vi "Write Pulse Recorder Configuration.vi"(8 "error in (no error)":errorcluster, 10 "Configuration":T1={"Post-trigger delay"=0.01, "Post-trigger duration"=0.1, "Rate"=1000000.0, "Ranges"=[10.0], "Re-name channels"=[], "Active channels"="0:1", "External clock"=FALSE} {"Rate" format="%#_8pHz"; "Post-trigger duration" format="%#_6ps"; "Post-trigger delay" format="%#_6ps"; "Ranges" format="%#_6pV"}, 11 "RP I-V in":refnum<class "RP I-V.lvclass">) -> (0 "error out":errorcluster, 3 "RP I-V out":refnum<class "RP I-V.lvclass">)   [LabVIEW 2021, in "RP I-V.lvclass"]
uses:
  RP I-V.lvclass
  NHMFL_Core/Libraries/Instruments/Pulse Driver/Pusle Driver Configuration.ctl
  RP I-V.lvclass/RP I-V.ctl
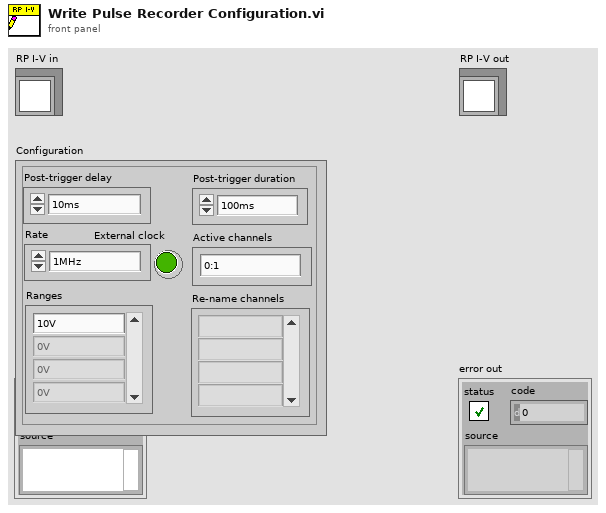
[diagram p1: front panel]
types:
  T1 = typedef "Pusle Driver Configuration.ctl" = cluster{"Post-trigger delay":dbl, "Post-trigger duration":dbl, "Rate":dbl, "Ranges":dbl[], "Re-name channels":string[], "Active channels":string, "External clock":bool}
  T2 = typedef "RP I-V Configuration.ctl" = cluster{"I-V parameters":T3, "Ranges":dbl[], "Post-trigger delay":dbl, "Post-trigger duration":dbl, "Output delay":dbl}
  T3 = typedef "I-V parameters.ctl" = cluster{"Start magnitude":dbl, "Magnitude increment":dbl, "End magnitude":dbl, "Ramp length":i32, "Top  length":i32, "Threshold ":dbl, "Processing delay":u16, "Valhalla range":dbl, "Interpolation":i32, "Stop after":u16, "Detector window":i32}
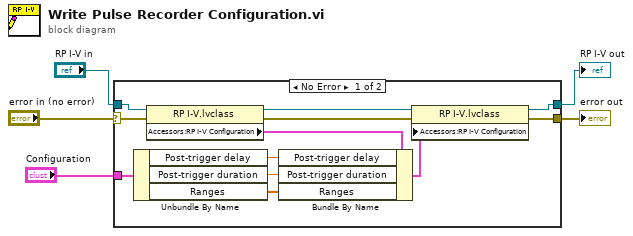
[diagram p0: block diagram]
diagram:
  n1 = case shown="No Error" "error in (no error)" {
    selector: "error in (no error)" -> [w10 w19]
    tunnel: [w12 w19] -> w2
    tunnel: "RP I-V in" -> [w15 w18]
    tunnel: "Configuration" -> [w9 _]
    tunnel: [w11 w18] -> w3
    frame No Error {
      n2 = Unbundle By Name(w9) -> ("Post-trigger delay"=w8:dbl, "Post-trigger duration"=w7:dbl, "Ranges"=w6:dbl[])
      n3 = property class="RP I-V.lvclass"(reference=w15, error in=w10) -> (reference out=w17:refnum<class "RP I-V.lvclass">, error out=w16:errorcluster, "Accessors:RP I-V Configuration"=w14:T2)
      n4 = Bundle By Name(cluster=w14, "Post-trigger delay"=w8, "Post-trigger duration"=w7, "Ranges"=w6) -> (w13:T2)
      n5 = property class="RP I-V.lvclass"(reference=w17, error in=w16, "Accessors:RP I-V Configuration"=w13) -> (reference out=w11:refnum<class "RP I-V.lvclass">, error out=w12:errorcluster)
    }
    frame Error {
    }
  }
  "error out" <- w2
  "RP I-V out" <- w3
